vi "Create Dir.vi"(8 "error in (no error)":errorcluster, 11 "appended path":path) -> (0 "error out":errorcluster, 3 "created path":path)   [LabVIEW 2014, in "lvprj2html.lvlib"]
uses:
  lvprj2html.lvlib
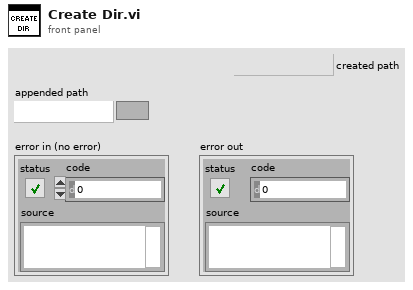
[diagram p1: front panel]
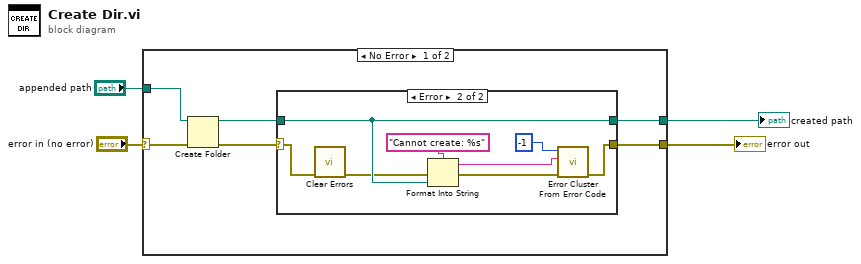
[diagram p0: block diagram]
diagram:
  n1 = case shown="No Error" "error in (no error)" {
    selector: "error in (no error)" -> [w9 w22]
    tunnel: "appended path" -> [w10 w21]
    tunnel: [w6 w22] -> w3
    tunnel: [w5 w21] -> w1
    frame No Error {
      n2 = Create Folder(path (use dialog)=w10, error in=w9) -> (created path=w7:path, error out=w8:errorcluster)  [unwired: 1 in, 1 out]
      n3 = case shown="Error" w8 {
        selector: w8 -> [w11 w14]
        tunnel: w7 -> [w12 w17]
        tunnel: [w12 w17] -> w5
        tunnel: [w11 w20] -> w6
        frame No Error {
        }
        frame Error {
          n4 = call <vilib>:"Clear Errors.vi"("error in (no error)"=w14) -> ("error out"=w13:errorcluster)  [unwired: 5 in, 1 out]
          n5 = Format Into String(format string="Cannot create: %s", error in=w13, w17) -> (resulting string=w16:string, error out=w15:errorcluster)  [unwired: 1 in]
          n6 = call <vilib>:"Error Cluster From Error Code.vi"("error in (no error)"=w15, "error message (\"\")"=w16, "error code (0)"=-1) -> ("error out"=w20:errorcluster)  [unwired: 6 in]
        }
      }
    }
    frame Error {
    }
  }
  "error out" <- w3
  "created path" <- w1
